vi "Close avi.vi"(8 "AVI refnum 2":T1, 9 "Camera 2?":bool, 10 "Save AVI?":bool, 11 "AVI refnum 1":T1) -> ()   [LabVIEW 2018]
uses:
  <vilib>/vision/Avi.llb/IMAQ AVI2 Refnum.ctl
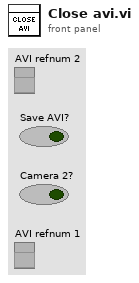
[diagram p1: front panel]
types:
  T1 = typedef "IMAQ AVI2 Refnum.ctl" = refnum<k20>
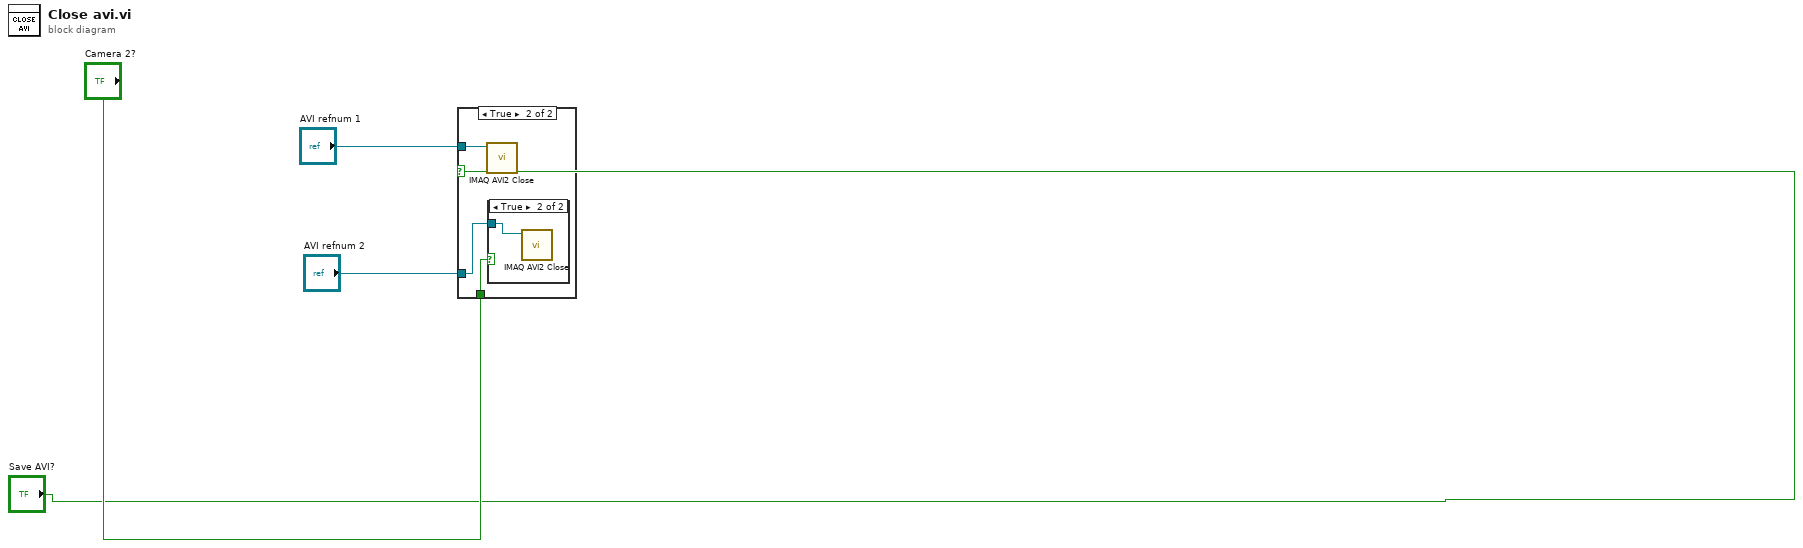
[diagram p0: block diagram]
diagram:
  n1 = case shown="True" "Save AVI?" {
    tunnel: "AVI refnum 1" -> [_ w7]
    tunnel: "AVI refnum 2" -> [_ w6]
    tunnel: "Camera 2?" -> [_ w5]
    frame False {
    }
    frame True {
      n2 = call "IMAQ AVI2 Close"("AVI Refnum"=w7) -> ()  [unwired: 10 in, 1 out]
      n3 = case shown="True" w5 {
        tunnel: w6 -> [_ w8]
        frame False {
        }
        frame True {
          n4 = call "IMAQ AVI2 Close"("AVI Refnum"=w8) -> ()  [unwired: 10 in, 1 out]
        }
      }
    }
  }
